vi "templogger.vi"(6 "error in (no error)":errorcluster, 8 "No. samples":i32, 9 "log to file":path=path "C:/Users/tuphe10-memsbuddy/Desktop/test temp AMI/test1.txt", 11 "VISA Cryocon":refnum<visa-resource-name>="GPIB1::12::INSTR") -> (4 "error out":errorcluster, 5 "VISA resource name":refnum<visa-resource-name>)   [LabVIEW 2013]
panel:
  in  "sample interval (sec)":dbl=0.2 format="%#_13g"
  out "Channel B":cluster{"X":dbl, "Y":dbl}[](graph)
  out "Channel A":cluster{"X":dbl, "Y":dbl}[](graph)
  out "Channel B (Vaporizer)":dbl format="%.2f"
  out "Channel A (Sample)":dbl format="%.2f"
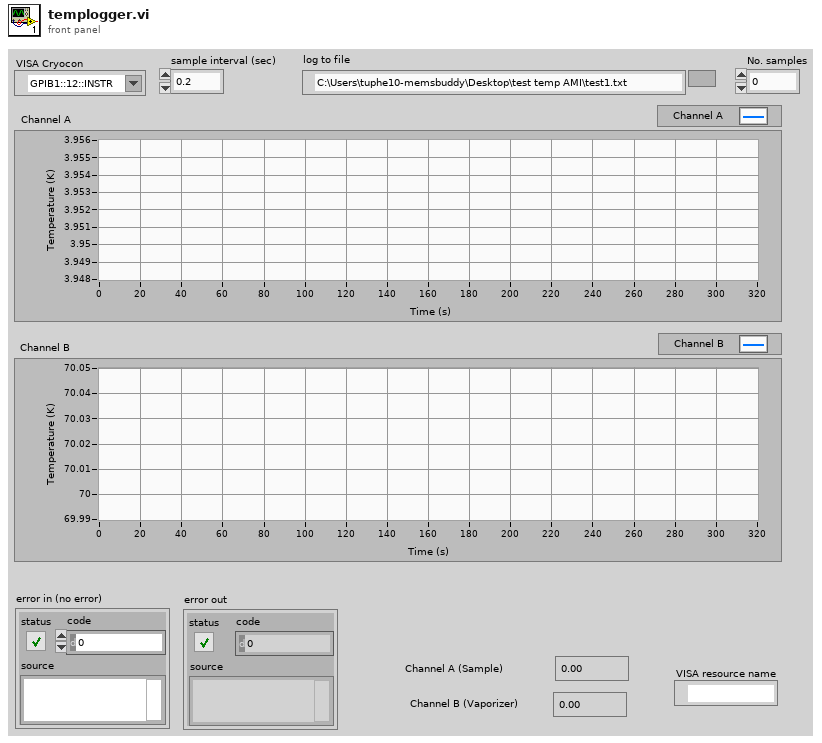
[diagram p1: front panel]
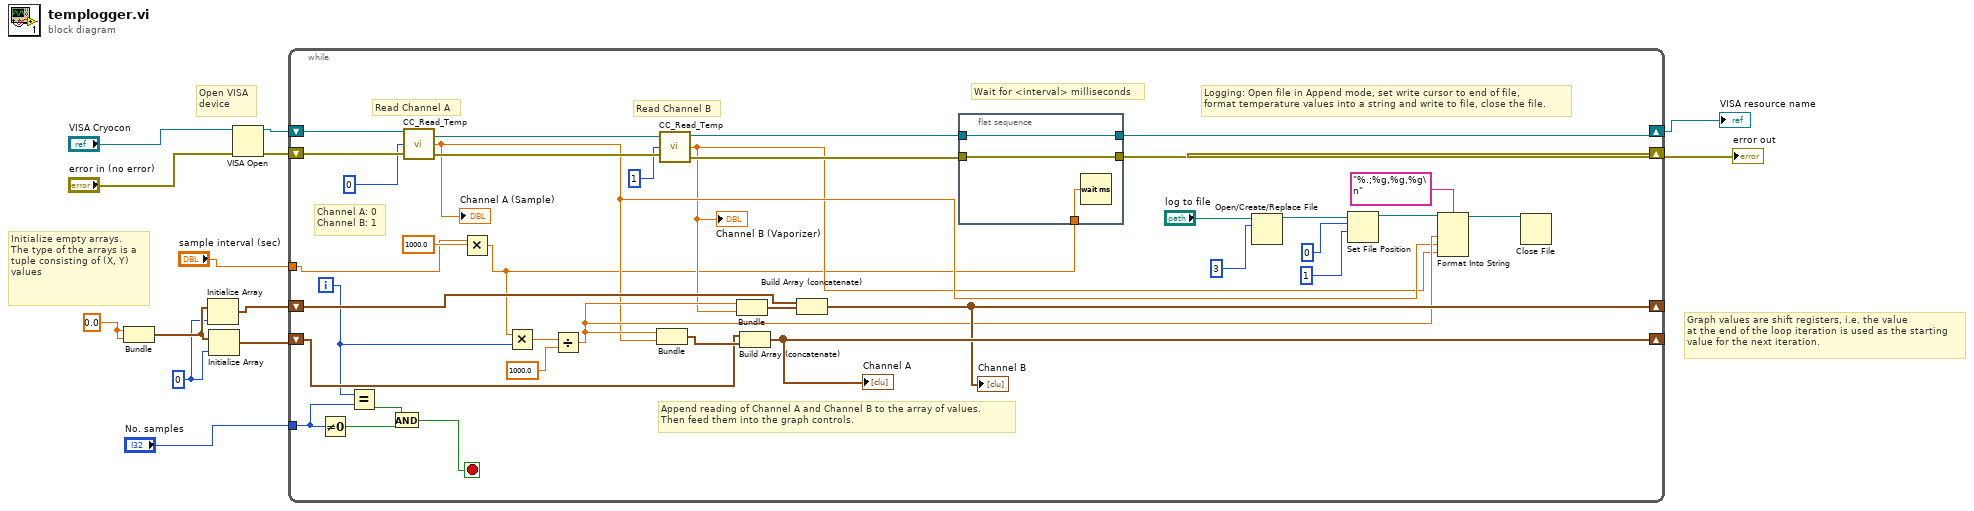
[diagram p0: block diagram]
diagram:
  w5 = 0
  w9 = 0.0
  # "Graph values are shift registers, i.e. the value\nat the end of the loop iteration is used as the starting\nvalue for the next iteration."
  # "Initialize empty arrays.\nThe type of the arrays is a tuple consisting of (X, Y) values"
  # "Open VISA\ndevice"
  n1 = Bundle(w9, w9) -> (w7:cluster{dbl, dbl})  [unwired: 1 in]
  n2 = Initialize Array(w7, w5) -> (w8:cluster{dbl, dbl}[])
  n3 = Initialize Array(w7, w5) -> (w6:cluster{dbl, dbl}[])
  n4 = VISA Open(error in (no error)="error in (no error)", VISA resource name="VISA Cryocon") -> (VISA resource name=w11:refnum<visa-resource-name>, error out=w10:errorcluster)  [unwired: 3 in]
  n5 = while {
    shift-right: [w47] -> w4
    shift-left: w10 -> [w49]
    shift-right: [w46] -> w2
    shift-left: w11 -> [w50]
    shift-right: [w36] -> _
    shift-left: w6 -> [w33]
    shift-right: [w35] -> _
    shift-left: w8 -> [w34]
    tunnel: "No. samples" -> [w19]
    tunnel: "sample interval (sec)" -> [w14]
    i -> [w18]
    stop <- w17 stop-if-true
    # "Logging: Open file in Append mode, set write cursor to end of file,\nformat temperature values into a string and write to file, close the file."
    # "Append reading of Channel A and Channel B to the array of values.\nThen feed them into the graph controls."
    # "Wait for <interval> milliseconds"
    # "Read Channel B"
    # "Read Channel A"
    # "Channel A: 0\nChannel B: 1"
    n6 = Not Equal To 0?(x=w19) -> (x != 0?=w21:bool)
    n7 = Equal?(x=w18, y=w19) -> (x = y?=w20:bool)
    n8 = And(x=w20, y=w21) -> (x .and. y?=w17:bool)
    n9 = call <userlib>:"CC_Read_Temp.vi"("error in (no error)"=w49, "Input"=0, "VISA In"=w50) -> ("error out"=w45:errorcluster, "Temperature"=w23:dbl, "VISA Out"=w42:refnum<visa-resource-name>)
    "Channel A (Sample)" <- w23
    n10 = Multiply(x=w14, y=1000.0) -> (x*y=w15:dbl)
    n11 = Multiply(x=w15, y=w18) -> (x*y=w40:dbl)
    n12 = Divide(x=w40, y=1000.0) -> (x/y=w24:dbl)
    n13 = Bundle(w24, "Temperature"=w23) -> (w38:cluster{dbl, "Temperature":dbl})  [unwired: 1 in]
    n14 = call <userlib>:"CC_Read_Temp.vi"("error in (no error)"=w45, "Input"=1, "VISA In"=w42) -> ("error out"=w44:errorcluster, "Temperature"=w22:dbl, "VISA Out"=w43:refnum<visa-resource-name>)
    "Channel B (Vaporizer)" <- w22
    n15 = Bundle(w24, "Temperature"=w22) -> (w37:cluster{dbl, "Temperature":dbl})  [unwired: 1 in]
    n16 = Build Array (concatenate)(w33, w38) -> (w36:cluster{dbl, "Temperature":dbl}[])
    "Channel A" <- w36
    n17 = Build Array (concatenate)(w34, w37) -> (w35:cluster{dbl, "Temperature":dbl}[])
    "Channel B" <- w35
    n18 = flat-sequence {
      tunnel: w43 -> [w52]
      tunnel: w44 -> [w53]
      tunnel: [w53] -> w47
      tunnel: [w52] -> w46
      tunnel: w15 -> [w51]
      frame #0 {
        n19 = Wait (ms)(milliseconds to wait=w51) -> ()  [unwired: 1 out]
      }
    }
    n20 = Open/Create/Replace File(file path (use dialog)="log to file", operation (0:open)=3) -> (refnum out=w30:refnum<file>)  [unwired: 4 in, 2 out]
    n21 = Set File Position(offset (in bytes) (0)=0, refnum=w30, from (0:start)=1) -> (refnum out=w29:refnum<file>)  [unwired: 1 in, 1 out]
    n22 = Format Into String(format string="%.;%g,%g,%g\n", initial string=w29, w24, w23, w22) -> (resulting string=w28:refnum<file>)  [unwired: 1 in, 1 out]
    n23 = Close File(refnum=w28) -> ()  [unwired: 1 in, 2 out]
  }
  "error out" <- w4
  "VISA resource name" <- w2
